vi "SetRCMFrameColor.vi"(4 "error in (no error)":errorcluster, 5 "Value":u32(colorbox), 6 "Container State":T2, 7 "Display State In":T1={"RCM File Path"=path "", "Left"=0, "Top"=0, "Font Name"="", "Font Size"=0, "Font Color"=0, "Separator Color"=9868950, "Frame Color"=9868950, "Overlay Color"=26367}) -> (0 "error out":errorcluster, 3 "Display State Out":T1={"RCM File Path"=path "", "Left"=0, "Top"=0, "Font Name"="", "Font Size"=0, "Font Color"=0, "Separator Color"=9868950, "Frame Color"=9868950, "Overlay Color"=26367})   [LabVIEW 2009, in "RCM.xctl"]
uses:
  RCM.xctl
  <vilib>/_xctls/Container State.ctl
  Ability/State_RCM.ctl
  <vilib>/_xctls/XControlSupport.lvlib
panel:
  # "Replace the Value Control below with a Control of desired type.\nDo not remove this Control or the others from the connector pane.\nDo not change the connector pane pattern.\nThe Value control should always be the third terminal from top on the input side in the connector pane."
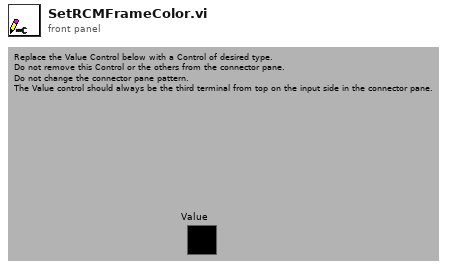
[diagram p1: front panel]
types:
  T1 = typedef "RCM.xctl/State_RCM.ctl" = cluster{"RCM File Path":path, "Left":u32, "Top":u32, "Font Name":string, "Font Size":i16, "Font Color":u32, "Separator Color":u32, "Frame Color":u32, "Overlay Color":u32}
  T2 = typedef "XControlSupport.lvlib/Container State.ctl" = cluster{"Indicator?":bool, "Run Mode?":bool, " Refnum":refnum<vi>}
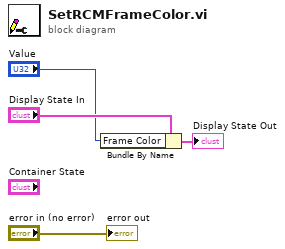
[diagram p0: block diagram]
diagram:
  n1 = Bundle By Name(cluster="Display State In", "Frame Color"="Value") -> (→"Display State Out":T1)
  "error out" <- "error in (no error)"
